vi "Split DMA by Direction.vi"(11 "DMA configuration array":T1[](array[typedef])) -> (1 "HostToTarget":T4[](array[typedef]) {"reservation info"."reserver ref in" format="%.0x"}, 3 "TargetToHost":T4[](array[typedef]) {"reservation info"."reserver ref in" format="%.0x"})   [LabVIEW 2016, in "FPGA Addon System Explorer.lvlib"]
uses:
  FPGA Addon System Explorer.lvlib
  DMA Reservation.ctl
  <vilib>/rvi/FIFO/Fifo_Types/Fifo_DMA_Config.ctl
  <vilib>/rvi/DataTransferAndStorage/Container/Common/niFpgaDataTypeControl.ctl
  <vilib>/rvi/ClientSDK/Core/ModuleGeneration/CommunicationInterfaceUtility/niFpgaDmaChannelImplementation.ctl
  reservation info.ctl
  <vilib>/NI Veristand/Custom Device API/Custom Device Item Ref.ctl
  <vilib>/NI VeriStand/Custom Device API/Custom Device API.lvlib
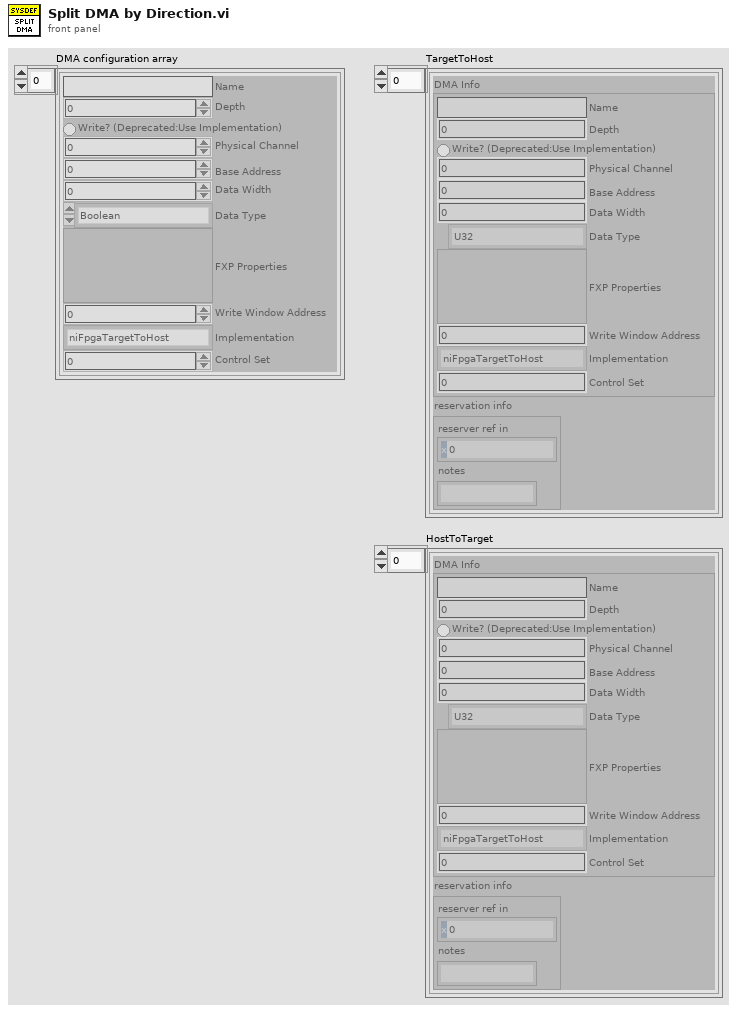
[diagram p1: front panel]
types:
  T1 = typedef "Fifo_DMA_Config.ctl" = cluster{"Name":string, "Depth":u32, "Write? (Deprecated:Use Implementation)":bool, "Physical Channel":u32, "Base Address":u32, "Data Width":u32, "Data Type":T2, "FXP Properties":variant, "Write Window Address":u32, "Implementation":T3, "Control Set":u32}
  T2 = typedef "niFpgaDataTypeControl.ctl" = enum32{"Boolean", "I8", "I16", "I32", "I64", "U8", "U16", "U32", "U64", "FXP", "CustomControl", "SGL"}
  T3 = typedef "niFpgaDmaChannelImplementation.ctl" = enum16{"niFpgaTargetToHost", "niFpgaHostToTarget", "niFpgaPeerToPeerWriter", "niFpgaPeerToPeerReader", "niCoreTargetToHost", "niCoreHostToTarget"}
  T4 = typedef "FPGA Addon System Explorer.lvlib/DMA Reservation.ctl" = cluster{"DMA Info":T1, "reservation info":T5}
  T5 = typedef "FPGA Addon System Explorer.lvlib/reservation info.ctl" = cluster{"reserver ref in":T6, "notes":string}
  T6 = typedef "Custom Device API.lvlib/Custom Device Item Ref.ctl" = u64
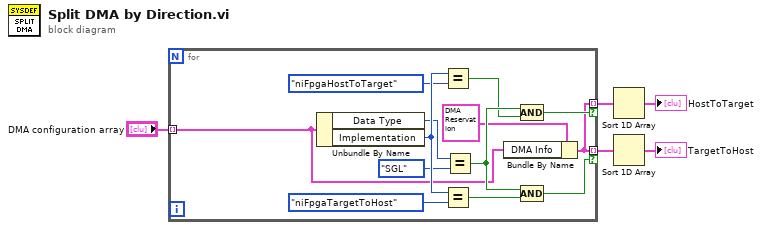
[diagram p0: block diagram]
diagram:
  n1 = for {
    tunnel: "DMA configuration array" -> [w7] mode=indexing
    tunnel: [w6] -> w1 mode=indexing if=w12
    tunnel: [w6] -> w3 mode=indexing if=w9
    n2 = Unbundle By Name(w7) -> ("Data Type"=w14:T2, "Implementation"=w17:T3)
    n3 = Equal?(x=w17, y=niFpgaDmaChannelImplementation."niFpgaHostToTarget") -> (x = y?=w10:bool)
    n4 = Equal?(x=w17, y=niFpgaDmaChannelImplementation."niFpgaTargetToHost") -> (x = y?=w15:bool)
    n5 = Equal?(x=w14, y=niFpgaDataTypeControl."SGL") -> (x = y?=w11:bool)
    n6 = Bundle By Name(cluster=T4 {"DMA Info"={"Name"="", "Depth"=0, "Write? (Deprecated:Use Implementation)"=FALSE, "Physical Channel"=0, "Base Address"=0, "Data Width"=0, "Data Type"=enum."U32", "FXP Properties"=variant, "Write Window Address"=0, "Implementation"=enum."niFpgaTargetToHost", "Control Set"=0}, "reservation info"={"reserver ref in"=0, "notes"=""}} ("DMA Reservation"), "DMA Info"=w7) -> (w6:T4)
    n7 = Compound Arithmetic op=AND(w11, w10) -> (w9:bool)
    n8 = Compound Arithmetic op=AND(w11, w15) -> (w12:bool)
  }
  n9 = Sort 1D Array(array=w3) -> (sorted array=→"HostToTarget":T4[])
  n10 = Sort 1D Array(array=w1) -> (sorted array=→"TargetToHost":T4[])
